vi "Create Body.vi"(0 "Name":string, 1 "Origin":refnum<vi>, 2 "Color":T1, 3 "Height":sgl, 4 "Radius":sgl) -> (7 "reference out":refnum<vi>, 8 "Head":refnum<vi>)   [LabVIEW 2010]
uses:
  <vilib>/picture/3D Picture Control/NI_3D Picture Control.lvlib
panel:
  out "Trans 3":refnum<vi>
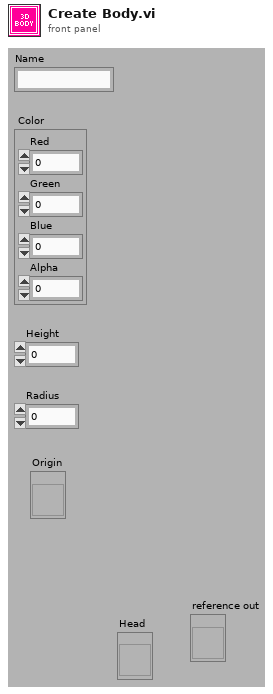
[diagram p1: front panel]
types:
  T1 = cluster{"Red":sgl, "Green":sgl, "Blue":sgl, "Alpha":sgl}
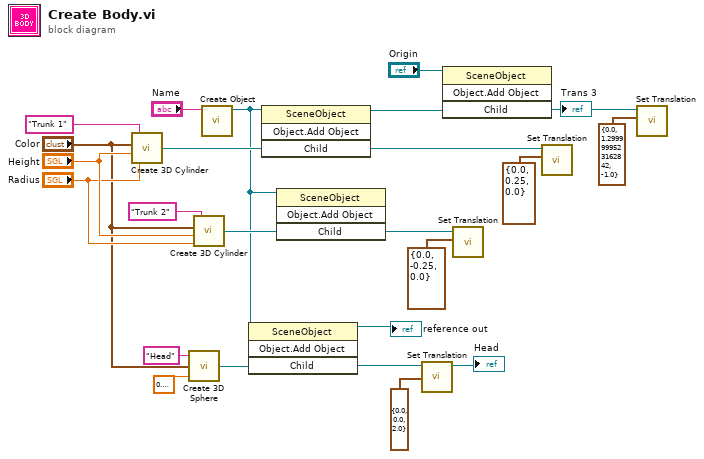
[diagram p0: block diagram]
diagram:
  n1 = call "Create 3D Cylinder.vi"("Radius"="Radius", "Height"="Height", "Color"="Color", "Name"="Trunk 1") -> ("Scene:New Object"=w22:refnum<vi>)
  n2 = call "Create 3D Sphere.vi"("Radius"=sgl 0.7, "Color"="Color", "Name"="Head") -> ("Scene:New Object"=w4:refnum<vi>)
  n3 = call "Create 3D Cylinder.vi"("Radius"="Radius", "Height"="Height", "Color"="Color", "Name"="Trunk 2") -> ("Scene:New Object"=w21:refnum<vi>)
  n4 = call <vilib>:"Create Object.vi"("Name"="Name") -> ("Scene:New Object"=w5:refnum<vi>)  [unwired: 9 in, 1 out]
  n5 = invoke class="SceneObject" method="Object.Add Object"(reference=w5, "Child"=w4) -> (reference out=→"reference out":refnum<vi>, "Child"=w3:refnum<vi>)  [unwired: 2 in, 2 out]
  n6 = invoke class="SceneObject" method="Object.Add Object"(reference=w5, "Child"=w22) -> (reference out=w16:refnum<vi>, "Child"=w10:refnum<vi>)  [unwired: 2 in, 2 out]
  n7 = invoke class="SceneObject" method="Object.Add Object"(reference=w5, "Child"=w21) -> ("Child"=w9:refnum<vi>)  [unwired: 2 in, 3 out]
  n8 = call <vilib>:"Set Translation.vi"("Translation"=cluster{"X":sgl, "Y":sgl, "Z":sgl} {"X"=0.0, "Y"=0.0, "Z"=2.0}, "Scene Object"=w3) -> ("Translated Object"=→"Head":refnum<vi>)  [unwired: 8 in, 1 out]
  n9 = invoke class="SceneObject" method="Object.Add Object"(reference="Origin", "Child"=w16) -> ("Child"=w11:refnum<vi>)  [unwired: 2 in, 3 out]
  "Trans 3" <- w11
  n10 = call <vilib>:"Set Translation.vi"("Translation"=cluster{"X":sgl, "Y":sgl, "Z":sgl} {"X"=0.0, "Y"=-0.25, "Z"=0.0}, "Scene Object"=w9) -> ()  [unwired: 8 in, 2 out]
  n11 = call <vilib>:"Set Translation.vi"("Translation"=cluster{"X":sgl, "Y":sgl, "Z":sgl} {"X"=0.0, "Y"=0.25, "Z"=0.0}, "Scene Object"=w10) -> ()  [unwired: 8 in, 2 out]
  n12 = call <vilib>:"Set Translation.vi"("Translation"=cluster{"X":sgl, "Y":sgl, "Z":sgl} {"X"=0.0, "Y"=1.3, "Z"=-1.0}, "Scene Object"=w11) -> ()  [unwired: 8 in, 2 out]
